vi "test.to.str.Time.vi"() -> ()   [LabVIEW 2020]
uses:
  fpga/orderbook.command.ctl
  fpga/orderbook.command.type.ctl
  fpganow.common.host.lvlib
  fpga/fpganow.common.fpga.lvlib
panel:
  out "Actual Out":string
  in  "Expected Out":string="(Time, 44700)"
  out "Passed?":bool
  in  "orderbook.command":T1={"type"=enum."Time", "side"=0, "orderId "=13758425324623625965, "quantity"=0, "symbol"=18369548393097576175, "price"=0, "executed.qty"=0, "canceled.qty"=0, "remaining.qty"=0, "seconds"=44700, "nanoseconds"=0, "Add"=FALSE, "Edit"=FALSE, "Remove"=FALSE, "seq no"=0, "recv.time"=0, "parse.time"=0} {"symbol" format="%.0x"; "orderId" format="%.0x"}
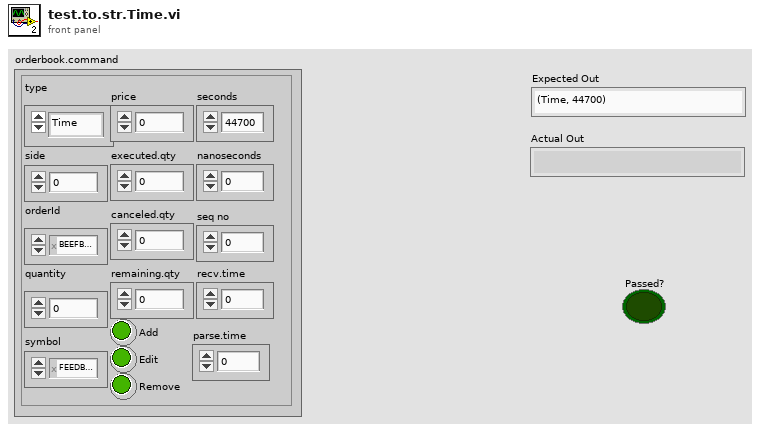
[diagram p1: front panel]
types:
  T1 = typedef "fpganow.common.fpga.lvlib/orderbook.command.ctl" = cluster{"type":T2, "side":u8, "orderId ":u64, "quantity":u32, "symbol":u64, "price":u64, "executed.qty":u32, "canceled.qty":u32, "remaining.qty":u32, "seconds":u64, "nanoseconds":u64, "Add":bool, "Edit":bool, "Remove":bool, "seq no":u32, "recv.time":u64, "parse.time":u64}
  T2 = typedef "fpganow.common.fpga.lvlib/orderbook.command.type.ctl" = enum8{"Time", "AddOrder", "OrderExecuted", "OrderExecutedAtPrice", "ReduceSize", "ModifyOrder", "DeleteOrder", "Get.Everything", "Get.All.Orders", "Get.Top"}
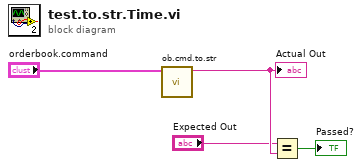
[diagram p0: block diagram]
diagram:
  n1 = call "ob.cmd.to.str.vi"("orderbook.command"="orderbook.command") -> ("string"=w3:string)  [unwired: 10 in]
  "Actual Out" <- w3
  n2 = Equal?(x="Expected Out", y=w3) -> (x = y?=→"Passed?":bool)
